vi "WL_XNET_GetDBC_WriteCluster.vi"(8 "err in":errorcluster caption="error", 10 "Signal Names":string[](array[string])=["LV_A_03_ETC_a_opCmd1_Error_Ack", "LV_A_03_ETC_a_opCmd1_Start_Stop", "LV_A_03_ETC_a_Speed_Set", "LV_A_11_HBV_a_Valve_Enable", "LV_A_11_HBV_a_Valve_Set", "LV_A_12_SIV_a_Valve_Enable", "LV_A_12_SIV_a_Valve_Set", "LV_A_13_SOV_a_Valve_Enable", "LV_A_13_SOV_a_Valve_Set", "LV_C_01_RF_a_FanSpeed", "LV_C_02_CP_a_RPM", "LV_E_74_ISO_a_Rq_D_IMC_STEST_SCR", "LV_E_75_HVP_a_Relais_Set", "LV_E_76_HVM_a_Relais_Set", "LV_H_31_OTV_a_Valve_Set", "LV_H_38_HSV_a_Valve_Set", "LV_H_42_HRB_a_FCCU_Spd_Rq", "LV_H_42_HRB_a_KNF_Speed_Rq", "LV_H_43_HDV_a_Dosing_Valve_Set", "LV_H_46_HRBo_a_Drain_Valve_Set", "LV_H_52_DV_a_Drain_Valve_Stack", "LV_H_53_PV_a_Purge_Valve_Stack", "LV_Testmode_Select", "S80_BP_s_Taster_Start_Status", "S80_BP_s_Taster_Stop_Status"], 11 "DBC_Settings_complete":T1={"ByteOrder"=[enum."Motorola", enum."Motorola"], "Type"=[], "Factor"=[1.0, 1.0], "Offset"=[0.0, 0.0], "Startbit"=[27, 43], "Length"=[16, 16], "Mux"=[FALSE, FALSE], "Name"=["", ""]} {"Offset" format="%.3f"; "Factor" format="%.3f"}) -> (0 "err out":errorcluster caption="error", 3 "DBC_Settings_clustered":T1={"ByteOrder"=[enum."Motorola", enum."Motorola"], "Type"=[], "Factor"=[1.0, 1.0], "Offset"=[0.0, 0.0], "Startbit"=[27, 43], "Length"=[16, 16], "Mux"=[FALSE, FALSE], "Name"=["", ""]} {"Offset" format="%.3f"; "Factor" format="%.3f"})   [LabVIEW 2021]
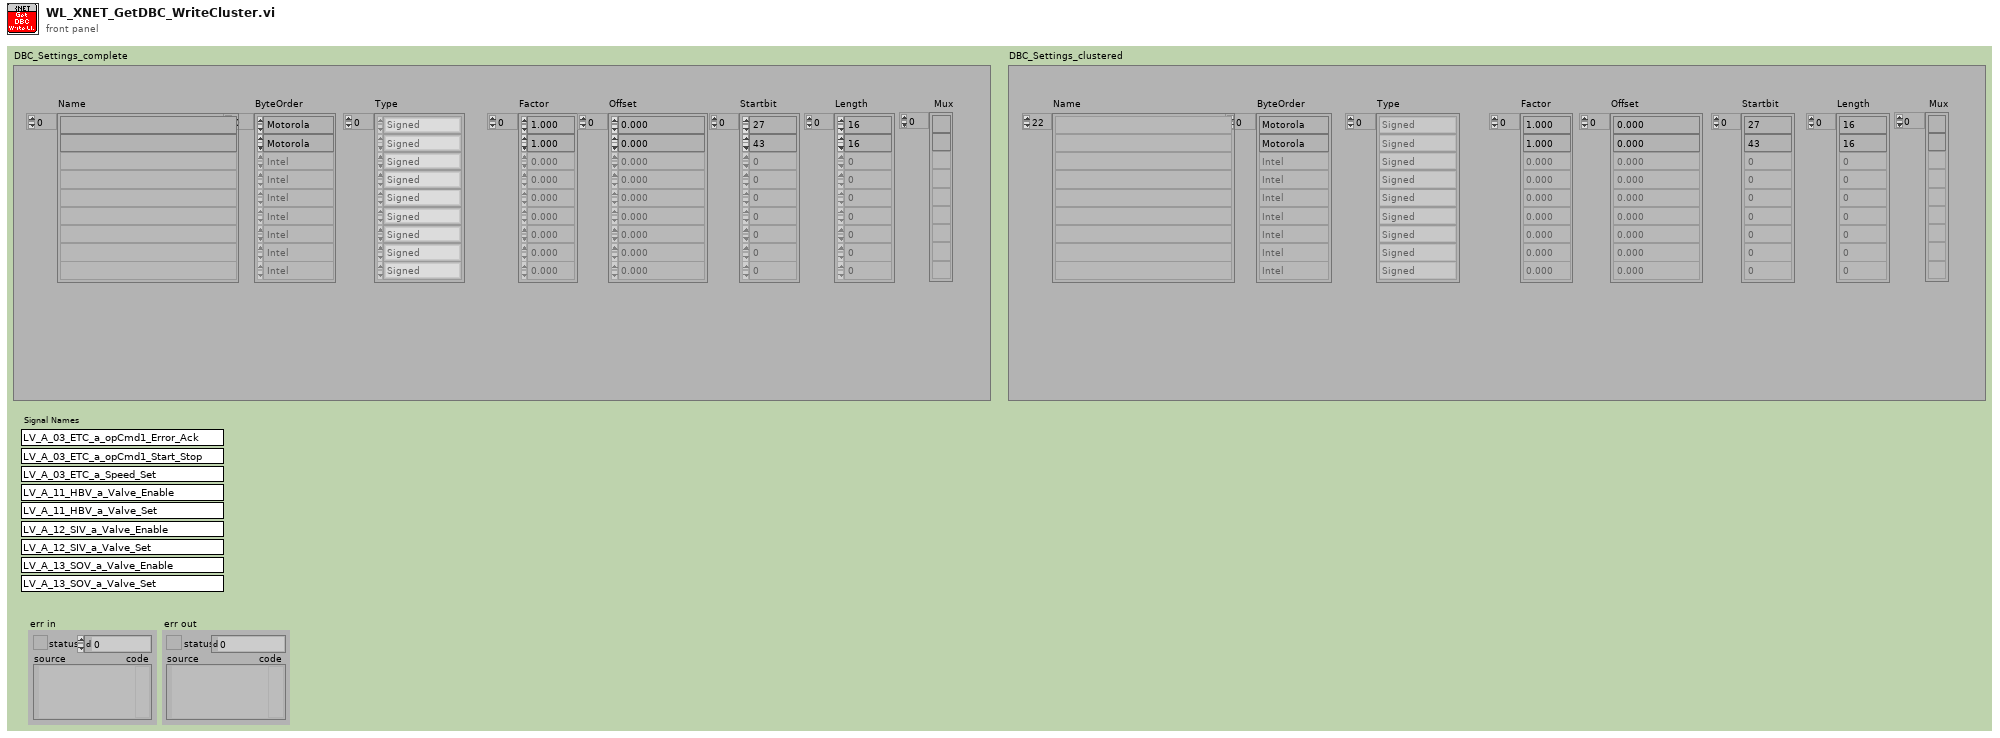
[diagram p1: front panel]
types:
  T1 = cluster{"ByteOrder":enum16{"Intel", "Motorola"}[], "Type":enum16{"Signed", "Unsigned", "IEEE Float", "Byte Array"}[], "Factor":dbl[], "Offset":dbl[], "Startbit":u32[], "Length":u32[], "Mux":bool[], "Name":string[]}
  T2 = enum16{"Signed", "Unsigned", "IEEE Float", "Byte Array"}[]
  T3 = enum16{"Signed", "Unsigned", "IEEE Float", "Byte Array"}
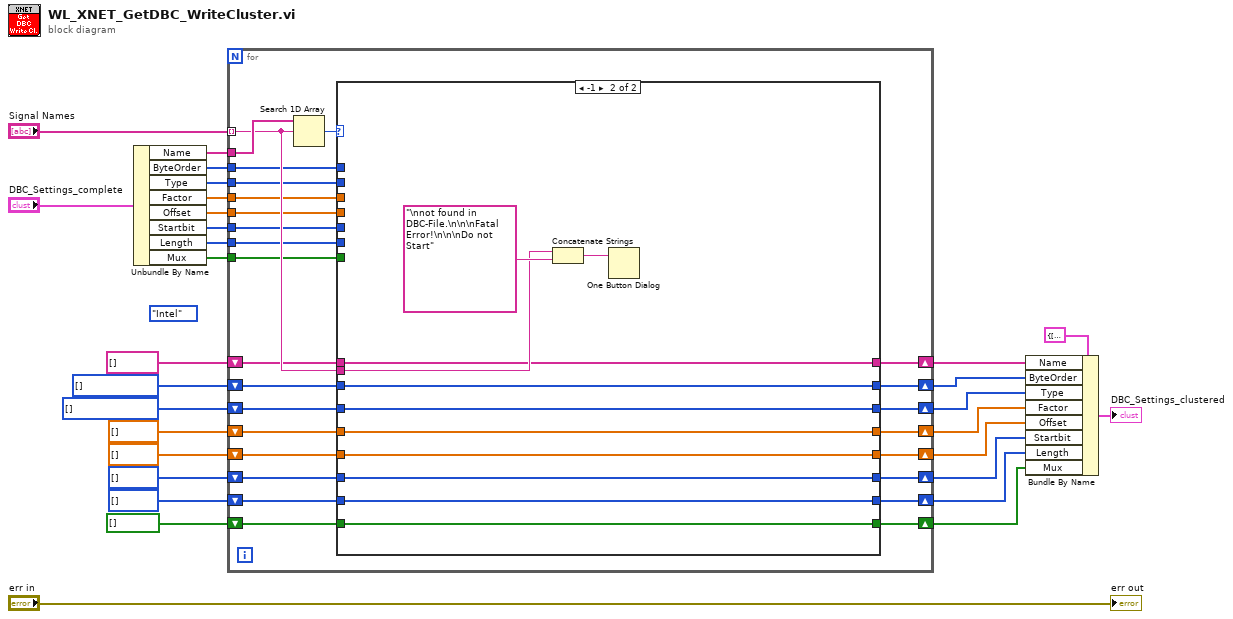
[diagram p0: block diagram]
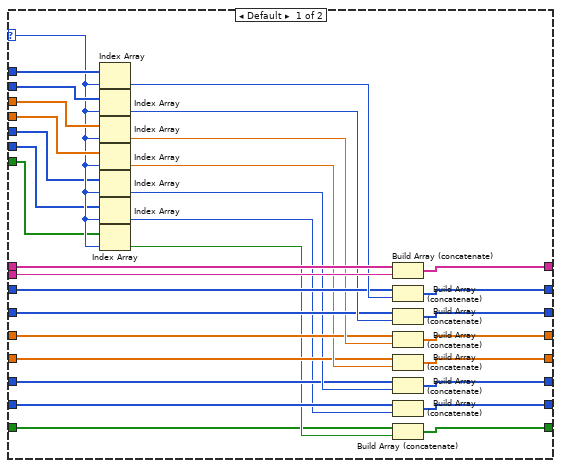
[diagram p2: hidden frame]
diagram:
  (unwired) enum16{"Intel", "Motorola"}."Intel" ("ByteAnordnung")
  w10 = T2 [] items=["Signed", "Unsigned", "IEEE Float", "Byte Array"] ("Type")
  w11 = enum16{"Intel", "Motorola"}[] [] items=["Intel", "Motorola"] ("ByteOrder")
  n1 = Unbundle By Name("DBC_Settings_complete") -> ("Name"=w26:string[], "ByteOrder"=w25:enum16{"Intel", "Motorola"}[], "Type"=w24:T2, "Factor"=w23:dbl[], "Offset"=w22:dbl[], "Startbit"=w21:u32[], "Length"=w20:u32[], "Mux"=w19:bool[])
  n2 = for {
    tunnel: "Signal Names" -> [w53] mode=indexing
    tunnel: w26 -> [w55]
    tunnel: w25 -> [w52]
    tunnel: w24 -> [w47]
    tunnel: w23 -> [w44]
    tunnel: w22 -> [w43]
    tunnel: w21 -> [w38]
    tunnel: w20 -> [w37]
    tunnel: w19 -> [w36]
    shift-right: [w50] -> w12
    shift-left: string[] [] ("Name") -> [w51]
    shift-right: [w48] -> w9
    shift-left: w11 -> [w49]
    shift-right: [w45] -> w8
    shift-left: w10 -> [w46]
    shift-right: [w41] -> w7
    shift-left: dbl[] [] ("Factor") -> [w42]
    shift-right: [w39] -> w6
    shift-left: dbl[] [] ("Offset") -> [w40]
    shift-right: [w32] -> w4
    shift-left: u32[] [] ("Startbit") -> [w35]
    shift-right: [w31] -> w3
    shift-left: u32[] [] ("Length") -> [w34]
    shift-right: [w30] -> w2
    shift-left: bool[] [] ("Mux") -> [w33]
    n3 = Search 1D Array(1D array=w55, element=w53) -> (index of element=w54:i32)  [unwired: 1 in]
    n4 = case shown="-1" w54 {
      selector: w54 -> [w68 _]
      tunnel: w53 -> [w85 w97]
      tunnel: w52 -> [w87 _]
      tunnel: w51 -> [w86 w93]
      tunnel: [w84 w93] -> w50
      tunnel: w49 -> [w82 w95]
      tunnel: [w81 w95] -> w48
      tunnel: w47 -> [w80 _]
      tunnel: w46 -> [w78 w94]
      tunnel: [w77 w94] -> w45
      tunnel: w44 -> [w76 _]
      tunnel: w43 -> [w75 _]
      tunnel: w42 -> [w73 w92]
      tunnel: [w72 w92] -> w41
      tunnel: w40 -> [w70 w91]
      tunnel: [w69 w91] -> w39
      tunnel: w38 -> [w67 _]
      tunnel: w37 -> [w66 _]
      tunnel: w36 -> [w65 _]
      tunnel: w35 -> [w63 w90]
      tunnel: w34 -> [w62 w89]
      tunnel: w33 -> [w59 w88]
      tunnel: [w58 w90] -> w32
      tunnel: [w57 w89] -> w31
      tunnel: [w56 w88] -> w30
      frame Default {
        n5 = Index Array(array=w87, index=w68) -> (element=w83:enum16{"Intel", "Motorola"})
        n6 = Index Array(array=w80, index=w68) -> (element=w79:T3)
        n7 = Index Array(array=w76, index=w68) -> (element=w74:dbl)
        n8 = Index Array(array=w75, index=w68) -> (element=w71:dbl)
        n9 = Index Array(array=w67, index=w68) -> (element=w64:u32)
        n10 = Index Array(array=w66, index=w68) -> (element=w61:u32)
        n11 = Index Array(array=w65, index=w68) -> (element=w60:bool)
        n12 = Build Array (concatenate)(w86, w85) -> (w84:string[])
        n13 = Build Array (concatenate)(w82, w83) -> (w81:enum16{"Intel", "Motorola"}[])
        n14 = Build Array (concatenate)(w78, w79) -> (w77:T2)
        n15 = Build Array (concatenate)(w73, w74) -> (w72:dbl[])
        n16 = Build Array (concatenate)(w70, w71) -> (w69:dbl[])
        n17 = Build Array (concatenate)(w63, w64) -> (w58:u32[])
        n18 = Build Array (concatenate)(w62, w61) -> (w57:u32[])
        n19 = Build Array (concatenate)(w59, w60) -> (w56:bool[])
      }
      frame -1 {
        n20 = Concatenate Strings(w97, "\nnot found in DBC-File.\n\n\nFatal Error!\n\n\nDo not Start" ("message")) -> (w96:string)
        n21 = One Button Dialog(message=w96) -> ()  [unwired: 1 in, 1 out]
      }
    }
  }
  n22 = Bundle By Name(cluster=T1 {"ByteOrder"=[], "Type"=[], "Factor"=[], "Offset"=[], "Startbit"=[], "Length"=[], "Mux"=[], "Name"=[]} ("DBC Settings"), "Name"=w12, "ByteOrder"=w9, "Type"=w8, "Factor"=w7, "Offset"=w6, "Startbit"=w4, "Length"=w3, "Mux"=w2) -> (→"DBC_Settings_clustered":T1)
  "err out" <- "err in"
